vi "Query Steps.vi"() -> ()   [LabVIEW 2024]
uses:
  9f6a4753-484f-4a8c-b075-228156ab4398.vi
  bc1a519a-6171-4a9d-bb0e-3749302a1243.vi
  <vilib>/Plug-In SDKs/Clients/Data Store V1/Data Store Client.lvlibp
panel:
  in  "odata query":string="$filter=contains(Name,'Voltage')"
  out "error out":errorcluster
  out "Filtered Steps":string[](array[string])
  out "All Steps":string[](array[string])
  # "Query Steps\n\nThis VI provides examples of querying Step items.\nRun Publish Data.vi to create data to query with this VI."
  # "Edit this odata query string and run this VI to change Filtered Steps below."
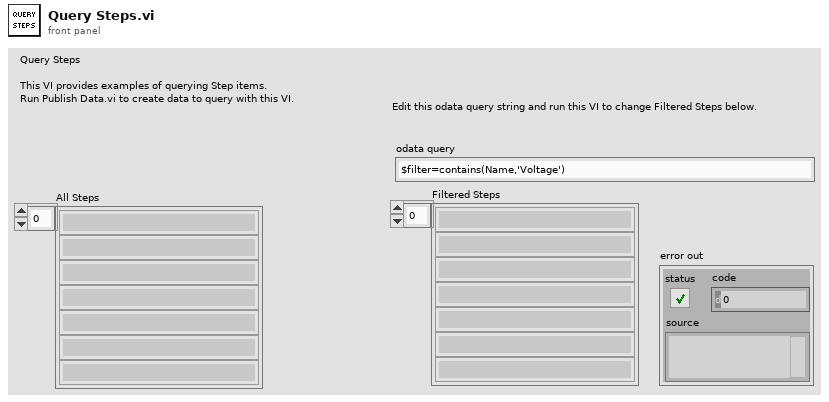
[diagram p1: front panel]
types:
  T1 = typedef "NI Metadata Types.lvlib/Step.ctl" = cluster{"step name":string, "step type":string, "start date time":timestamp, "end date time":timestamp, "notes":string, "step id":string, "parent step id":string, "test result id":string, "test id":string, "link":string, "extensions":T2[], "schema id":string}
  T2 = typedef "NI Metadata Types.lvlib/Extension.ctl" = cluster{"name":string, "value":string}
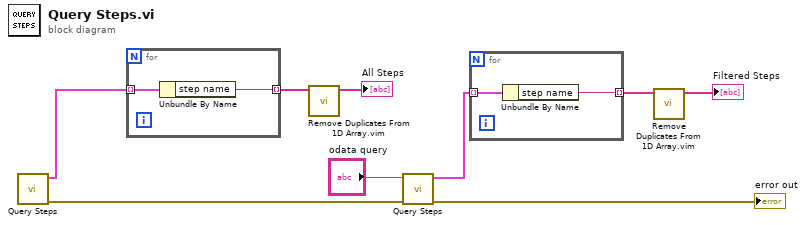
[diagram p0: block diagram]
diagram:
  n1 = call <vilib>:"Query Steps.vi"() -> ("error out"=w8:errorcluster, "steps"=w7:T1[])  [unwired: 10 in]
  n2 = for {
    tunnel: w7 -> [w11] mode=indexing
    tunnel: [w10] -> w4 mode=indexing
    n3 = Unbundle By Name(w11) -> ("step name"=w10:string)
  }
  n4 = call "Remove Duplicates From 1D Array.vim"("array"=w4) -> ("array with duplicates removed"=→"All Steps":string[])  [unwired: 10 in]
  n5 = call <vilib>:"Query Steps.vi"("error in"=w8, "odata query"="odata query") -> ("error out"=→"error out":errorcluster, "steps"=w6:T1[])  [unwired: 8 in]
  n6 = for {
    tunnel: w6 -> [w13] mode=indexing
    tunnel: [w12] -> w2 mode=indexing
    n7 = Unbundle By Name(w13) -> ("step name"=w12:string)
  }
  n8 = call "Remove Duplicates From 1D Array.vim"("array"=w2) -> ("array with duplicates removed"=→"Filtered Steps":string[])  [unwired: 10 in]
